vi "audio_tvPIP.vi"(8 "error in (no error)":errorcluster) -> (0 "error out":errorcluster, 2 "AUDIO-19":string, 3 "TV-20":string)   [LabVIEW 2018]
uses:
  Global_1259.vi
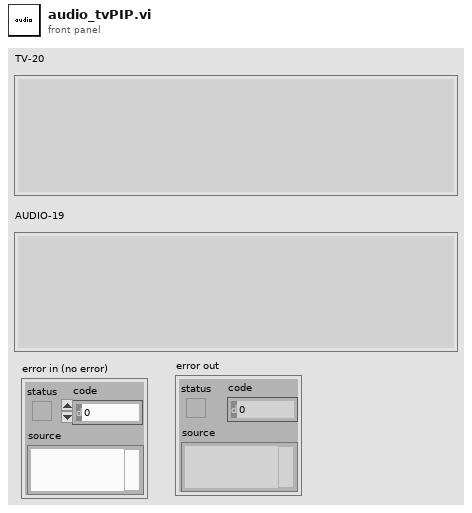
[diagram p1: front panel]
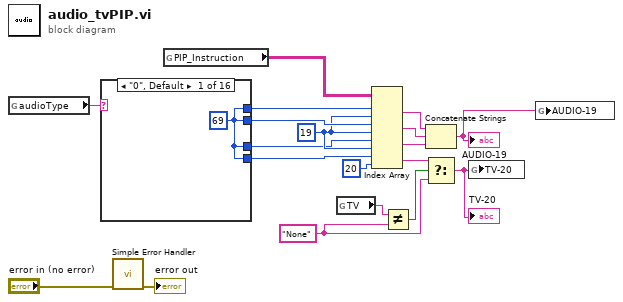
[diagram p0: block diagram]
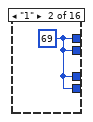
[diagram p2: hidden frame]
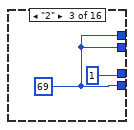
[diagram p3: hidden frame]
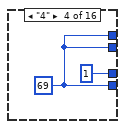
[diagram p4: hidden frame]
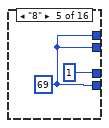
[diagram p5: hidden frame]
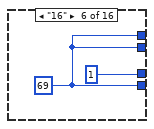
[diagram p6: hidden frame]
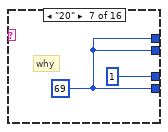
[diagram p7: hidden frame]
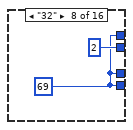
[diagram p8: hidden frame]
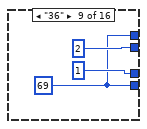
[diagram p9: hidden frame]
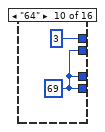
[diagram p10: hidden frame]
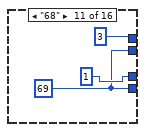
[diagram p11: hidden frame]
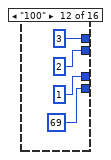
[diagram p12: hidden frame]
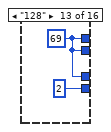
[diagram p13: hidden frame]
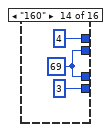
[diagram p14: hidden frame]
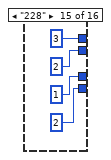
[diagram p15: hidden frame]
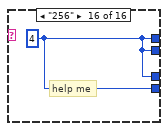
[diagram p16: hidden frame]
diagram:
  w7 = 19
  w19 = "None"
  n1 = global read "Global_1259.vi" "audioType"() -> (w13:string)
  n2 = case shown="\"0\", Default" w13 {
    tunnel: [w20 w21 w22 w24 w26 w28 w30 w32 w34 3 3 3 w46 4 3 w55] -> w18
    tunnel: [w20 w21 1 1 1 1 1 w32 1 w37 1 1 w46 w48 1 w55] -> w5
    tunnel: [w20 w21 w22 w24 w26 w28 w30 2 2 w37 w39 2 w46 w48 2 w55] -> w10
    tunnel: [w20 w21 w22 w24 w26 w28 w30 w32 w34 w37 w39 69 2 3 2 w55] -> w3
    frame "0", Default {
      w20 = 69
    }
    frame "1" {
      w21 = 69
    }
    frame "2" {
      w22 = 69
    }
    frame "4" {
      w24 = 69
    }
    frame "8" {
      w26 = 69
    }
    frame "16" {
      w28 = 69
    }
    frame "20" {
      w30 = 69
      # "why"
    }
    frame "32" {
      w32 = 69
    }
    frame "36" {
      w34 = 69
    }
    frame "64" {
      w37 = 69
    }
    frame "68" {
      w39 = 69
    }
    frame "100" {
    }
    frame "128" {
      w46 = 69
    }
    frame "160" {
      w48 = 69
    }
    frame "228" {
    }
    frame "256" {
      w55 = 4
      # "help me"
    }
  }
  n3 = call <vilib>:"Simple Error Handler.vi"("error in (no error)"="error in (no error)") -> ("error out"=→"error out":errorcluster)  [unwired: 4 in, 4 out]
  n4 = global read "Global_1259.vi" "PIP_Instruction"() -> (w15:string[][])
  n5 = global read "Global_1259.vi" "TV"() -> (w17:string)
  n6 = Index Array(array=w15, index (row) #1=w18, index (col) #1=w7, index (row) #2=w10, index (col) #2=w7, index (row) #3=w5, index (col) #3=w7, index (row) #4=w3, index (col) #4=20) -> (element #1=w8:string, element #2=w2:string, element #3=w1:string, element #4=w6:string)
  n7 = Not Equal?(x=w17, y=w19) -> (x != y?=w14:bool)
  n8 = Concatenate Strings(w8, w2, w1) -> (w9:string)
  "AUDIO-19" <- w9
  n9 = Select(t=w6, s=w14, f=w19) -> (s? t:f=w16:string)
  "TV-20" <- w16
  n10 = global write "Global_1259.vi" "TV-20"(w16) -> ()
  n11 = global write "Global_1259.vi" "AUDIO-19"(w9) -> ()
